vi "data to acc_gyro_enc.vi"(0 "byte array":u8[](array[numeric]), 1 "gyro range (deg/s)":dbl=250.0, 2 "accel range (m/s2)":dbl=8.0) -> (3 "acc gyro data":T1)   [LabVIEW 2012]
uses:
  acc_gyro_enc_data.ctl
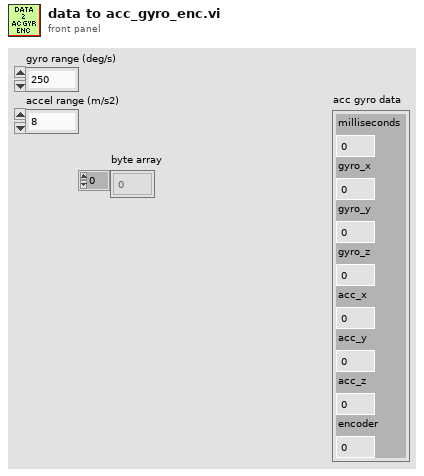
[diagram p1: front panel]
types:
  T1 = typedef "acc_gyro_enc_data.ctl" = cluster{"milliseconds":u64, "gyro_x":dbl, "gyro_y":dbl, "gyro_z":dbl, "acc_x":dbl, "acc_y":dbl, "acc_z":dbl, "encoder":i32}
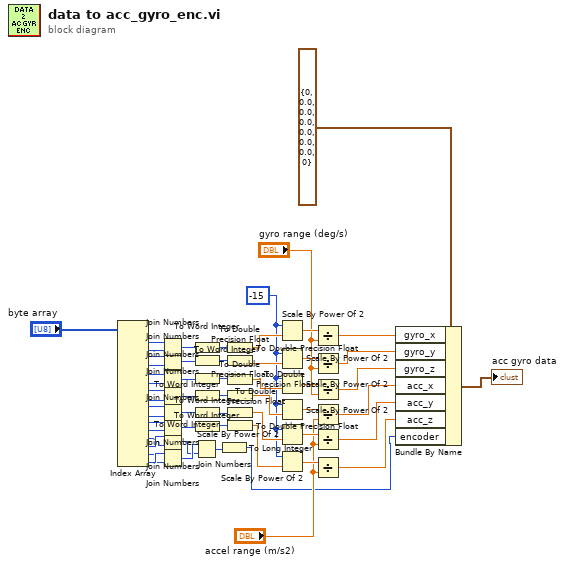
[diagram p0: block diagram]
diagram:
  w25 = -15
  n1 = Index Array(array="byte array") -> (element #1=w55:u8, element #2=w54:u8, element #3=w53:u8, element #4=w52:u8, element #5=w51:u8, element #6=w50:u8, element #7=w49:u8, element #8=w48:u8, element #9=w47:u8, element #10=w46:u8, element #11=w45:u8, element #12=w44:u8, element #13=w3:u8, element #14=w4:u8, element #15=w5:u8, element #16=w6:u8)  [unwired: 16 in]
  n2 = Join Numbers(hi=w55, lo=w54) -> ((hi.lo)=w43:u16)
  n3 = Join Numbers(hi=w53, lo=w52) -> ((hi.lo)=w42:u16)
  n4 = Join Numbers(hi=w51, lo=w50) -> ((hi.lo)=w41:u16)
  n5 = Join Numbers(hi=w49, lo=w48) -> ((hi.lo)=w40:u16)
  n6 = Join Numbers(hi=w47, lo=w46) -> ((hi.lo)=w39:u16)
  n7 = Join Numbers(hi=w45, lo=w44) -> ((hi.lo)=w38:u16)
  n8 = Join Numbers(hi=w4, lo=w3) -> ((hi.lo)=w1:u16)
  n9 = Join Numbers(hi=w6, lo=w5) -> ((hi.lo)=w2:u16)
  n10 = To Word Integer(number=w43) -> (16bit integer=w37:i16)
  n11 = To Word Integer(number=w42) -> (16bit integer=w36:i16)
  n12 = To Word Integer(number=w41) -> (16bit integer=w35:i16)
  n13 = To Word Integer(number=w40) -> (16bit integer=w34:i16)
  n14 = To Word Integer(number=w39) -> (16bit integer=w33:i16)
  n15 = To Word Integer(number=w38) -> (16bit integer=w32:i16)
  n16 = Join Numbers(hi=w2, lo=w1) -> ((hi.lo)=w8:u32)
  n17 = To Long Integer(number=w8) -> (32bit integer=w7:i32)
  n18 = To Double Precision Float(number=w37) -> (double precision float=w31:dbl)
  n19 = To Double Precision Float(number=w36) -> (double precision float=w30:dbl)
  n20 = To Double Precision Float(number=w35) -> (double precision float=w29:dbl)
  n21 = To Double Precision Float(number=w34) -> (double precision float=w28:dbl)
  n22 = To Double Precision Float(number=w33) -> (double precision float=w27:dbl)
  n23 = To Double Precision Float(number=w32) -> (double precision float=w26:dbl)
  n24 = Scale By Power Of 2(n=w25, x=w31) -> (x*2^n=w24:dbl)
  n25 = Scale By Power Of 2(n=w25, x=w30) -> (x*2^n=w23:dbl)
  n26 = Scale By Power Of 2(n=w25, x=w29) -> (x*2^n=w21:dbl)
  n27 = Scale By Power Of 2(n=w25, x=w28) -> (x*2^n=w22:dbl)
  n28 = Scale By Power Of 2(n=w25, x=w27) -> (x*2^n=w20:dbl)
  n29 = Scale By Power Of 2(n=w25, x=w26) -> (x*2^n=w19:dbl)
  n30 = Divide(x=w24, y="gyro range (deg/s)") -> (x/y=w16:dbl)
  n31 = Divide(x=w23, y="gyro range (deg/s)") -> (x/y=w15:dbl)
  n32 = Divide(x=w21, y="gyro range (deg/s)") -> (x/y=w14:dbl)
  n33 = Divide(x=w22, y="accel range (m/s2)") -> (x/y=w13:dbl)
  n34 = Divide(x=w20, y="accel range (m/s2)") -> (x/y=w12:dbl)
  n35 = Divide(x=w19, y="accel range (m/s2)") -> (x/y=w11:dbl)
  n36 = Bundle By Name(cluster=T1 {"milliseconds"=0, "gyro_x"=0.0, "gyro_y"=0.0, "gyro_z"=0.0, "acc_x"=0.0, "acc_y"=0.0, "acc_z"=0.0, "encoder"=0} ("acc gyro data"), "gyro_x"=w16, "gyro_y"=w15, "gyro_z"=w14, "acc_x"=w13, "acc_y"=w12, "acc_z"=w11, "encoder"=w7) -> (→"acc gyro data":T1)
